vi "A串口LABVIEW.vi"() -> (6 "产品ID":string)   [LabVIEW 2011]
panel:
  in  "布尔":bool
  out "错误输出":errorcluster
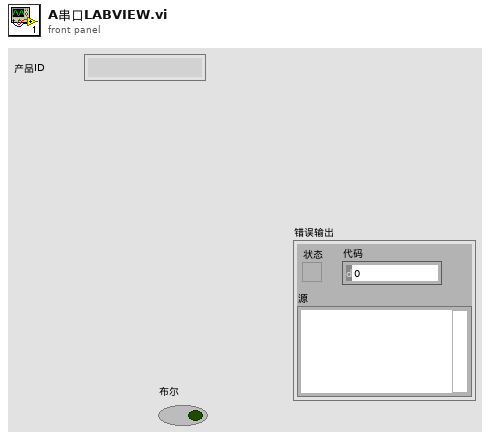
[diagram p1: front panel]
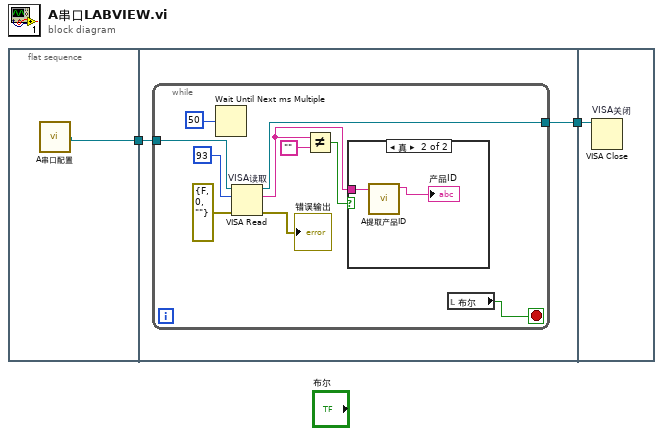
[diagram p0: block diagram]
diagram:
  n1 = flat-sequence {
    tunnel: [w3] -> w2
    tunnel: w2 -> [w5]
    tunnel: [w4] -> w1
    tunnel: w1 -> [w18]
    frame #0 {
      n2 = call "A串口配置.vi"() -> ("VISA resource name out"=w3:refnum<visa-resource-name>)  [unwired: 5 in]
    }
    frame #1 {
      n3 = while {
        tunnel: w5 -> [w15]
        tunnel: [w10] -> w4
        stop <- w6 stop-if-true
        n4 = Wait Until Next ms Multiple(millisecond multiple=u32 50 ("毫秒倍数")) -> ()  [unwired: 1 out]
        n5 = VISA Read "VISA读取"(VISA resource name=w15, byte count=u32 93 ("字节总数"), error in (no error)=errorcluster {"status"=FALSE, "code"=0, "source"=""} ("错误输入（无错误）")) -> (VISA resource name out=w10:refnum<visa-resource-name>, read buffer=w11:string, error out=→"错误输出":errorcluster)  [unwired: 1 out]
        n6 = Not Equal?(x=w11, y="") -> (x != y?=w12:bool)
        n7 = case shown="真" w12 {
          tunnel: w11 -> [_ w17]
          frame False {
          }
          frame True {
            n8 = call "A提取产品ID.vi"("字符串"=w17) -> ("产品ID"=→"产品ID":string)  [unwired: 10 in]
          }
        }
        n9 = local read "布尔"() -> (w6:bool)
      }
    }
    frame #2 {
      n10 = VISA Close "VISA关闭"(VISA resource name=w18) -> ()  [unwired: 1 in, 1 out]
    }
  }
